vi "Query Multi Eval Meas List ES Flatness MaxR Limit Check Results.vi"(7 "Result Type (Current)":i32(ring) items=["Current", "Average", "Extreme"], 8 "error in (no error)":errorcluster, 9 "Range (1)":T1=1, 10 "Instance (1)":T2=1, 11 "VISA resource name":refnum<visa-resource-name>) -> (0 "error out":errorcluster, 1 "ES Flatness MaxR Limit Check Results":i32[](array[numeric]), 2 "Reliability":i32, 3 "VISA resource name out":refnum<visa-resource-name>)   [LabVIEW 2015, in "Rohde&Schwarz CMXP NR FR2 Measurement.lvlib"]
doc: "Returns the limit check results for equalizer spectrum flatness single value results (maximum within a range) for all measured list mode segments.\n\nAttributes:\nRSCMXPNRFR2M_ATTR_QUERY_MULTI_EVAL_MEASUREMENT_LIST_ESF_MAXR_AVERAGE_LIMIT_CHECK_RESULTS\nRSCMXPNRFR2M_ATTR_QUERY_MULTI_EVAL_MEASUREMENT_LIST_ESF_MAXR_CURRENT_LIMIT_CHECK_RESULTS\nRSCMXPNRFR2M_ATTR_QUERY_MULTI_EVAL_MEASUREMENT_LIST_ESF_MAXR_EXTREME_LIMIT_CHECK_RESULTS\n\nRemote-control commands:\nCALCulate:NRMMw:MEAS<i>:MEValuation:LIST:ESFLatness:MAXR<no>:AVERage?\nCALCulate:NRMMw:MEAS<i>:MEValuation:LIST:ESFLatness:MAXR<no>:CURRent?\nCALCulate:NRMMw:MEAS<i>:MEValuation:LIST:ESFLatness:MAXR<no>:EXTReme?"
uses:
  <instrlib>/Rohde&Schwarz CMXP NR FR2 Measurement/Rohde&Schwarz CMXP NR FR2 Measurement.lvlib
  <instrlib>/Rohde&Schwarz CMXP NR FR2 Measurement/Private/_Instance.ctl
  <instrlib>/Rohde&Schwarz CMXP NR FR2 Measurement/Private/_Range.ctl
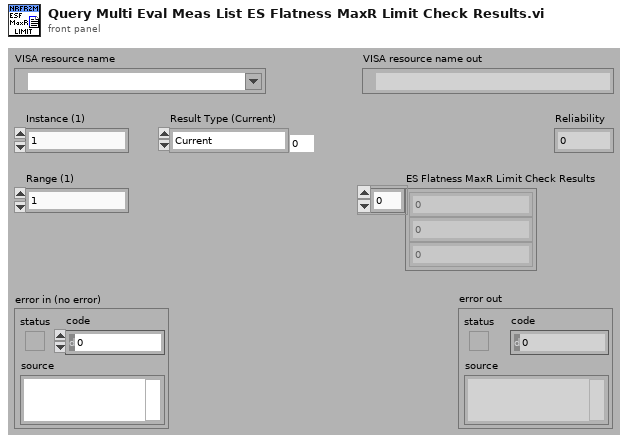
[diagram p1: front panel]
types:
  T1 = typedef "Rohde&Schwarz CMXP NR FR2 Measurement.lvlib/_Range.ctl" = i32
  T2 = typedef "Rohde&Schwarz CMXP NR FR2 Measurement.lvlib/_Instance.ctl" = i32
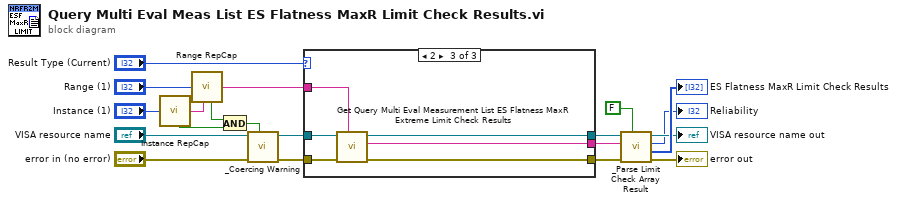
[diagram p0: block diagram]
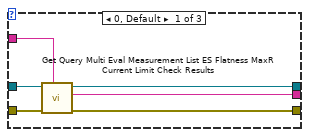
[diagram p2: hidden frame]
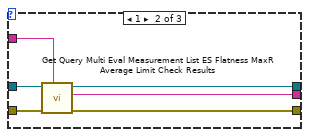
[diagram p3: hidden frame]
diagram:
  n1 = call <instrlib>:"Instance RepCap.vi"("Instance In"="Instance (1)") -> ("In Range?"=w18:bool, "RepCap Identifier Out"=w1:string)  [unwired: 1 in]
  n2 = call <instrlib>:"Range RepCap.vi"("Range In"="Range (1)", "RepCap String In (\"\")"=w1) -> ("In Range?"=w20:bool, "RepCap Identifier Out"=w11:string)
  n3 = And(x=w20, y=w18) -> (x .and. y?=w19:bool)
  n4 = call <instrlib>:"_Coercing Warning.vi"("In Range?"=w19, "error in (no error)"="error in (no error)", "VISA resource name"="VISA resource name") -> ("error out"=w13:errorcluster, "VISA resource name out"=w12:refnum<visa-resource-name>)  [unwired: 7 in]
  n5 = case shown="2" "Result Type (Current)" {
    tunnel: w13 -> [w26 w32 w38]
    tunnel: w12 -> [w25 w31 w37]
    tunnel: [w24 w30 w36] -> w10
    tunnel: [w23 w29 w35] -> w9
    tunnel: [w22 w28 w34] -> w8
    tunnel: w11 -> [w21 w27 w33]
    frame 0, Default {
      n6 = call "Get Query Multi Eval Measurement List ES Flatness MaxR Current Limit Check Results"("Repeated Capabilities"=w21, "error in (no error)"=w26, "instrument handle"=w25) -> ("error out"=w24:errorcluster, "Query Multi Eval Measurement List ES Flatness MaxR Current Limit Check Results"=w23:string, "instrument handle out"=w22:refnum<visa-resource-name>)  [unwired: 6 in]
    }
    frame 1 {
      n7 = call "Get Query Multi Eval Measurement List ES Flatness MaxR Average Limit Check Results"("Repeated Capabilities"=w27, "error in (no error)"=w32, "instrument handle"=w31) -> ("error out"=w30:errorcluster, "Query Multi Eval Measurement List ES Flatness MaxR Average Limit Check Results"=w29:string, "instrument handle out"=w28:refnum<visa-resource-name>)  [unwired: 6 in]
    }
    frame 2 {
      n8 = call "Get Query Multi Eval Measurement List ES Flatness MaxR Extreme Limit Check Results"("Repeated Capabilities"=w33, "error in (no error)"=w38, "instrument handle"=w37) -> ("error out"=w36:errorcluster, "Query Multi Eval Measurement List ES Flatness MaxR Extreme Limit Check Results"=w35:string, "instrument handle out"=w34:refnum<visa-resource-name>)  [unwired: 6 in]
    }
  }
  n9 = call <instrlib>:"_Parse Limit Check Array Result.vi"("error in (no error)"=w10, "Input String"=w9, "VISA resource name"=w8, "Out of tolerance? (F)"=FALSE) -> ("error out"=→"error out":errorcluster, "Results"=→"ES Flatness MaxR Limit Check Results":i32[], "Reliability"=→"Reliability":i32, "VISA resource name out"=→"VISA resource name out":refnum<visa-resource-name>)  [unwired: 3 in]
